vi "Get Data.vi"(8 "error in (no error)":errorcluster, 11 "Cap Bank Controller in":refnum<class "Cap Bank Interface.lvclass">) -> (0 "error out":errorcluster, 3 "Cap Bank Controller out":refnum<class "Cap Bank Interface.lvclass">)   [LabVIEW 2015, in "Cap Bank Interface.lvclass"]
uses:
  Cap Bank Interface.lvclass
  <vilib>/ActorFramework/Actor/Actor.lvclass/Actor.ctl
  Cap Bank Interface.lvclass/Cap Bank Interface.ctl
  Cap Bank Server Messages/Recieve Bank Shot Result Msg/Recieve Bank Shot Result Msg.lvclass/Recieve Bank Shot Result Msg.ctl
  <vilib>/ActorFramework/Message Enqueuer/Message Enqueuer.lvclass/Message Enqueuer.ctl
  Mag Lab Measure Controller Messages/Log Status Update Msg/Log Status Update Msg.lvclass/Log Status Update Msg.ctl
  <vilib>/ActorFramework/Message Enqueuer/Enqueue.vi
  <vilib>/ActorFramework/Message Priority Queue/Priority Enqueue.vi
  Cap Bank Server Messages/Recieve Bank Shot Result Msg/Recieve Bank Shot Result Msg.lvclass
  Mag Lab Measure Controller Messages/Log Status Update Msg/Log Status Update Msg.lvclass
  <vilib>/ActorFramework/Actor/Actor.lvclass
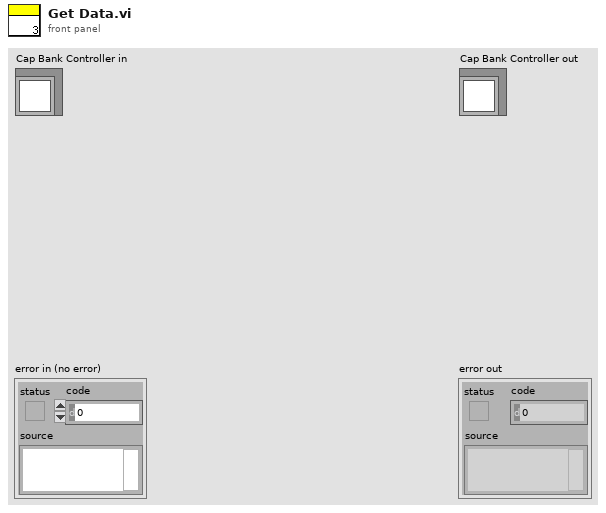
[diagram p1: front panel]
types:
  T1 = typedef "OPC connections.ctl" = cluster{"Data received":refnum<k13>, "Data Ready":refnum<k13>, "Message":refnum<k13>}
  T2 = typedef "Shot data.ctl" = cluster{"Shot number":i32, "Time":timestamp, "Magnet ID":string, "User":string, "Cell number":i32, "Requested field":dbl, "Field direction":string, "Number of bank frames":i32, "Crowbar resistance, mOhm":dbl, "Magnet resistance, mOhm":dbl, "Charger voltage, kV":dbl, "Frame voltage, kV":dbl}
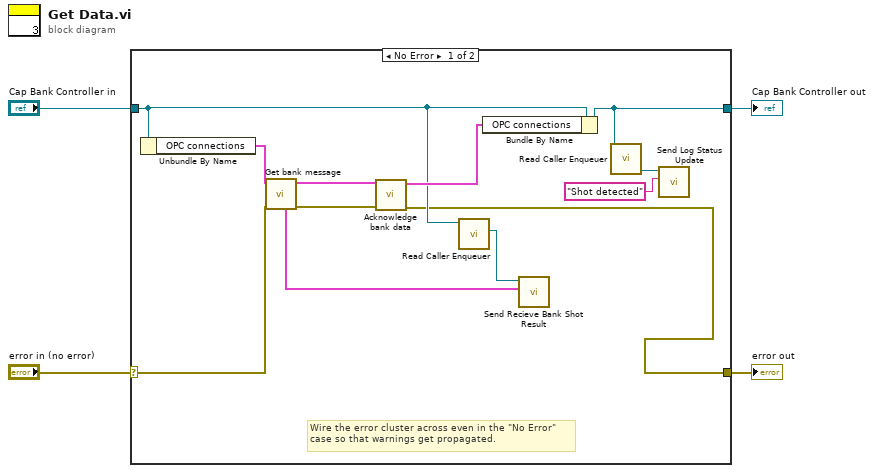
[diagram p0: block diagram]
diagram:
  n1 = case shown="No Error" "error in (no error)" {
    selector: "error in (no error)" -> [w15 w18]
    tunnel: [w8 w18] -> w3
    tunnel: [w5 w17] -> w1
    tunnel: "Cap Bank Controller in" -> [w12 w17]
    frame No Error {
      # "Wire the error cluster across even in the \"No Error\"\ncase so that warnings get propagated."
      n2 = Unbundle By Name(w12) -> ("OPC connections"=w16:T1)
      n3 = call "Get bank message.vi"("error IO"=w15, "OPC connections"=w16) -> ("error out"=w11:errorcluster, "OPC connections out"=w14:T1, "Shot data"=w9:T2)  [unwired: 4 in, 3 out]
      n4 = call "Acknowledge bank data.vi"("error in"=w11, "OPC connections"=w14) -> ("error out"=w8:errorcluster, "OPC connections out"=w13:T1)  [unwired: 7 in, 1 out]
      n5 = call <vilib>:"Read Caller Enqueuer.vi"("Actor"=w12) -> ("Caller Enqueuer"=w10:refnum<class "Message Enqueuer.lvclass">)  [unwired: 10 in]
      n6 = Bundle By Name(cluster=w12, "OPC connections"=w13) -> (w5:refnum<class "Cap Bank Interface.lvclass">)
      n7 = call "Send Recieve Bank Shot Result.vi"("Shot data"=w9, "Message Enqueuer"=w10) -> ()  [unwired: 8 in, 2 out]
      n8 = call <vilib>:"Read Caller Enqueuer.vi"("Actor"=w5) -> ("Caller Enqueuer"=w7:refnum<class "Message Enqueuer.lvclass">)  [unwired: 10 in]
      n9 = call "Send Log Status Update.vi"("Status"="Shot detected", "Message Enqueuer"=w7) -> ()  [unwired: 8 in, 2 out]
    }
    frame Error {
    }
  }
  "error out" <- w3
  "Cap Bank Controller out" <- w1
